vi "Write Filter Configuration Array.vi"(10 "Filter Configuration Array":refnum<class "Base Filter.lvclass">[](array[class]), 11 "Main Display in":refnum<class "Main Display.lvclass">) -> (3 "Main Display out":refnum<class "Main Display.lvclass">)   [LabVIEW 2016, in "Assert API Components.lvlib" / "Assert Display.lvlib" / "Main Display.lvlib" / "Main Display.lvclass"]
uses:
  Main Display.lvclass
  Assert API Components/Filter Configurations/Base Filter.lvclass
  Main Display.lvclass/Main Display.ctl
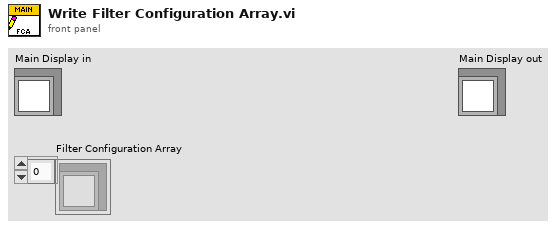
[diagram p1: front panel]
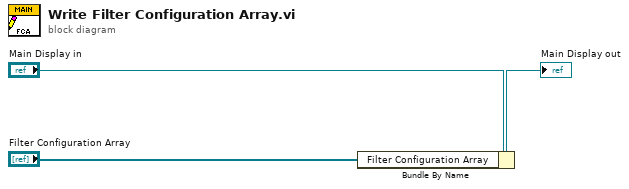
[diagram p0: block diagram]
diagram:
  n1 = Bundle By Name(cluster="Main Display in", "Filter Configuration Array"="Filter Configuration Array") -> (→"Main Display out":refnum<class "Main Display.lvclass">)
